vi "Find Tests from Path.vi"(8 "error in (no error)":errorcluster, 10 "Test File Path":path, 11 "Execution UI in":refnum<class "Execution UI.lvclass">) -> (0 "error out":errorcluster, 3 "Execution UI out":refnum<class "Execution UI.lvclass">)   [LabVIEW 2020, in "Execution UI.lvclass"]
uses:
  Execution UI.lvclass
  C:/git/astemes-lunit/source/User Interface/Process/Process.lvclass
  Process/Process.lvclass/Process.ctl
  Execution UI.lvclass/Execution UI.ctl
  Process/Process.lvclass
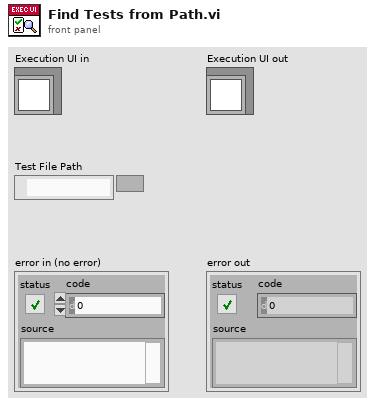
[diagram p1: front panel]
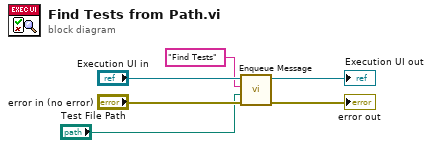
[diagram p0: block diagram]
diagram:
  n1 = call "Enqueue Message.vi"("error in (no error)"="error in (no error)", "Message Data"="Test File Path", "Message"="Find Tests", "Process In"="Execution UI in") -> ("error out"=→"error out":errorcluster, "Process Out"=→"Execution UI out":refnum<class "Execution UI.lvclass">)  [unwired: 6 in]
